vi "SafeParser_Integer.vi"(5 "Maximum":i32, 7 "Minimum":i32, 9 "Array Index":i32, 11 "String Array":string[](array[string])) -> (0 "Error Out":errorcluster, 3 "Typecast  Value":i32)   [LabVIEW 2019]
doc: "This VI is configured for polymorphic use and takes in an array of strings and converts one of those strings (specified by an index) to an integer. Error checking is performed including checking for acceptable data ranges. This VI is intended for use for the FRC 4265 autonomous parameter strings."
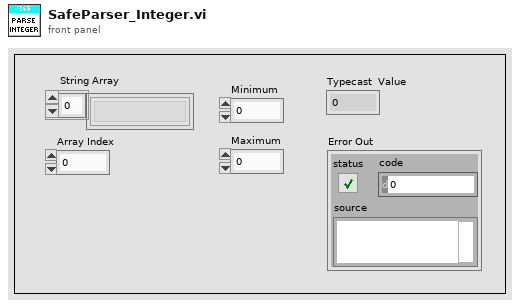
[diagram p1: front panel]
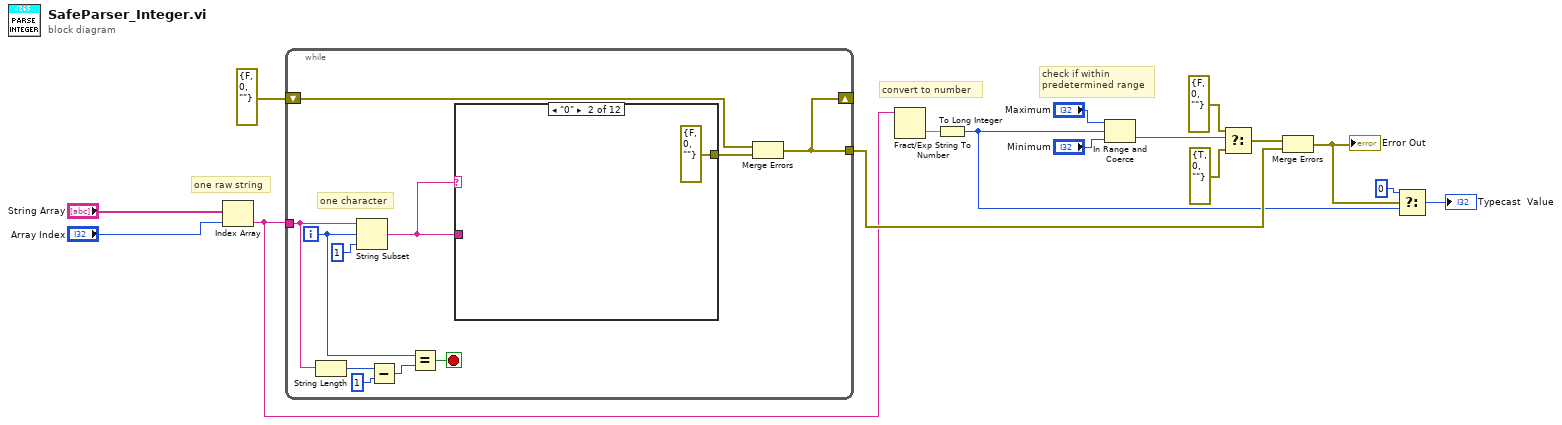
[diagram p0: block diagram]
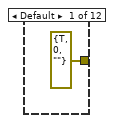
[diagram p2: hidden frame]
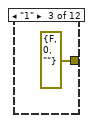
[diagram p3: hidden frame]
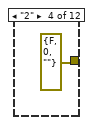
[diagram p4: hidden frame]
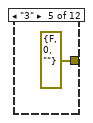
[diagram p5: hidden frame]
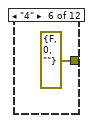
[diagram p6: hidden frame]
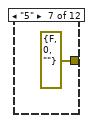
[diagram p7: hidden frame]
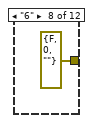
[diagram p8: hidden frame]
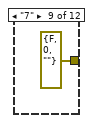
[diagram p9: hidden frame]
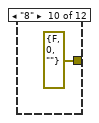
[diagram p10: hidden frame]
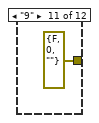
[diagram p11: hidden frame]
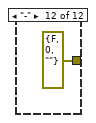
[diagram p12: hidden frame]
diagram:
  # "convert to number"
  # "check if within\npredetermined range"
  # "one raw string"
  n1 = Index Array(array="String Array", index="Array Index") -> (element=w7:string)
  n2 = while {
    tunnel: w7 -> [w26]
    shift-right: [w17] -> _
    shift-left: errorcluster {"status"=FALSE, "code"=0, "source"=""} ("error constant") -> [w18]
    tunnel: [w17] -> w8
    i -> [w23]
    stop <- w25 stop-if-true
    # "one character"
    n3 = String Length(string=w26) -> (length=w22:i32)
    n4 = String Subset(string=w26, offset (0)=w23, length (rest)=1) -> (substring=w24:string)
    n5 = Subtract(x=w22, y=1) -> (x-y=w20:i32)
    n6 = Equal?(x=w23, y=w20) -> (x = y?=w25:bool)
    n7 = case shown="\"0\"" w24 {
      tunnel: w24 -> [_ _ _ _ _ _ _ _ _ _ _ _]
      tunnel: [errorcluster {"status"=TRUE, "code"=0, "source"=""} ("error constant") errorcluster {"status"=FALSE, "code"=0, "source"=""} ("error constant") errorcluster {"status"=FALSE, "code"=0, "source"=""} ("error constant") errorcluster {"status"=FALSE, "code"=0, "source"=""} ("error constant") errorcluster {"status"=FALSE, "code"=0, "source"=""} ("error constant") errorcluster {"status"=FALSE, "code"=0, "source"=""} ("error constant") errorcluster {"status"=FALSE, "code"=0, "source"=""} ("error constant") errorcluster {"status"=FALSE, "code"=0, "source"=""} ("error constant") errorcluster {"status"=FALSE, "code"=0, "source"=""} ("error constant") errorcluster {"status"=FALSE, "code"=0, "source"=""} ("error constant") errorcluster {"status"=FALSE, "code"=0, "source"=""} ("error constant") errorcluster {"status"=FALSE, "code"=0, "source"=""} ("error constant")] -> w19
      frame Default {
      }
      frame "0" {
      }
      frame "1" {
      }
      frame "2" {
      }
      frame "3" {
      }
      frame "4" {
      }
      frame "5" {
      }
      frame "6" {
      }
      frame "7" {
      }
      frame "8" {
      }
      frame "9" {
      }
      frame "-" {
      }
    }
    n8 = Merge Errors(w18, w19) -> (w17:errorcluster)
  }
  n9 = Fract/Exp String To Number(string=w7) -> (number=w5:dbl)  [unwired: 3 in, 1 out]
  n10 = To Long Integer(number=w5) -> (32bit integer=w2:i32)
  n11 = In Range and Coerce(upper limit="Maximum", x=w2, lower limit="Minimum") -> (In Range?=w12:bool)  [unwired: 1 out]
  n12 = Select(t=errorcluster {"status"=FALSE, "code"=0, "source"=""} ("error constant"), s=w12, f=errorcluster {"status"=TRUE, "code"=0, "source"=""} ("error constant")) -> (s? t:f=w9:errorcluster)
  n13 = Merge Errors(w9, w8) -> (w6:errorcluster)
  "Error Out" <- w6
  n14 = Select(t=0, s=w6, f=w2) -> (s? t:f=→"Typecast  Value":i32)
